vi "WeDo-PyBD.vi"() -> ()   [LabVIEW 2016]
uses:
  VIs/uPythonX/uPythonX.xctl
panel:
  in  "WeDo":T1(xcontrol)={"VISA Refnum in"="ASRL23::INSTR", "Python Code"="import machine, utime\n\ntx = machine.Pin('Y1', machine.Pin.OUT)\nrx = machine.Pin('Y2', machine.Pin.IN)\ntx.value(b'\\x00')\nutime.sleep_ms(500)\ntx.value(1)\n\nuart = machine.UART(6)\nuart.init(baudrate=2400, bits=8, parity=None, stop=1)\n\nuart.write(0)\nuart.write(b'\\x40\\x23\\x9C')\nuart.write(b'\\x49\\x00\\x00\\xB6')\nuart.write(b'\\x46\\x00\\xB9')\nuart.write(b'\\x5A\\x60\\x00\\x09\\x00\\xCC')\nuart.write(b'\\x5F\\x01\\x00\\x00\\x00\\x01\\x00\\x00\\x00\\xA0')\nuart.write(b'\\x98\\x00\\x4C\\x69\\x67\\x68\\x74\\x00\\x00\\x00\\x39')\nuart.write(b'\\x90\\x80\\x01\\x00\\x03\\x00\\xED')\nuart.write(b'\\x04')\n"}
  # "Blue"
  # "Green"
  # "Yellow"
  # "Red"
  # "Orange"
  # "Magenta"
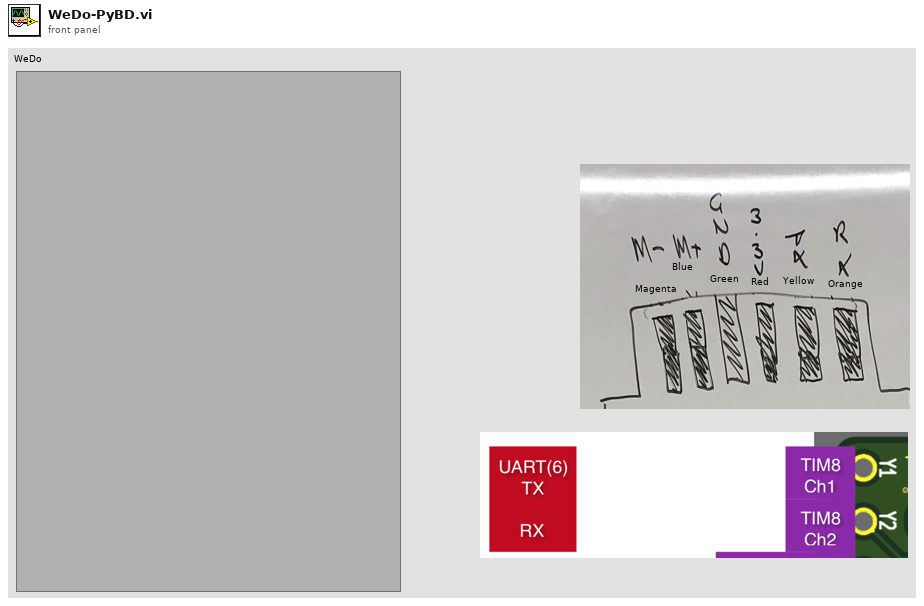
[diagram p1: front panel]
types:
  T1 = cluster{"VISA Refnum in":refnum<visa-resource-name>, "Python Code":string}
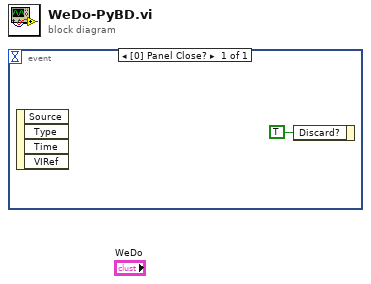
[diagram p0: block diagram]
diagram:
  n1 = event shown="[0] Panel Close?" {
    selector: _ -> [_]
    dyn-events: _ -> [_]
    timeout: _ -> [_]
    event Panel Close? {
      n2 = event-data() -> ()  [unwired: 1 in, 4 out]
      n3 = event-data("Discard?"=TRUE) -> ()  [unwired: 1 in, 1 out]
    }
  }
